vi "edit io channel.vi"(6 "user event":T2, 8 "error in":errorcluster, 9 "line":T1, 10 "engine configuration in":refnum<class "engine configuration.lvclass">, 11 "EthernetIP configuration in":refnum<class "EthernetIP configuration.lvclass">) -> (0 "error out":errorcluster, 2 "engine configuration out":refnum<class "engine configuration.lvclass">, 3 "EthernetIP configuration out":refnum<class "EthernetIP configuration.lvclass">)   [LabVIEW 2013, in "EthernetIP editor node.lvclass"]
uses:
  EthernetIP editor node.lvclass
  <vilib>/CEF_TreeControl/Node/UserEventRef.ctl
  <vilib>/CEF_TreeControl/Controls/EventCluster.ctl
  <vilib>/NI/Module Execution Interface/Engine Configuration/engine configuration.lvclass
  <vilib>/NI/TBM Modules/Ethernet IP/configuration/EthernetIP configuration.lvclass
  table line.ctl
  <vilib>/NI/TBM Modules/Ethernet IP/channel/EthernetIP Channel.lvclass
  <vilib>/NI/Tag Bus Module Framework/root configuration/TBM configuration.lvclass/TBM configuration.ctl
  <vilib>/NI/Tag Bus/tag/tag descriptor.lvclass/tag descriptor.ctl
  <vilib>/NI/Tag Bus Module Framework/root configuration/create GUID.vi
  <vilib>/CEF_TreeControl/NISE_CEF_TreeControl.lvlib
  <vilib>/NI/Tag Bus/tag/tag descriptor.lvclass
  <vilib>/NI/Tag Bus Module Framework/root configuration/TBM configuration.lvclass
  <vilib>/CEF_TreeControl/Node/NISE_CEF_Node.lvclass
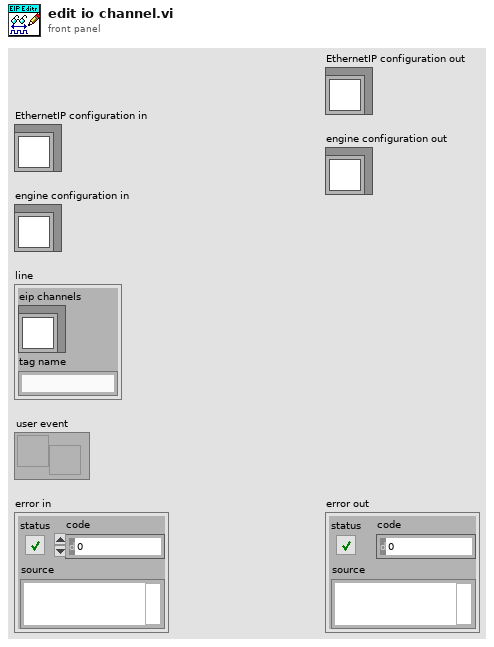
[diagram p1: front panel]
types:
  T1 = typedef "EthernetIP editor node.lvclass/table line.ctl" = cluster{"eip channels":refnum<class "EthernetIP Channel.lvclass">, "tag name":string}
  T2 = typedef "NISE_CEF_Node.lvclass/UserEventRef.ctl" = refnum<user-event>
  T3 = typedef "NISE_CEF_TreeControl.lvlib/EventCluster.ctl" = cluster{"command":string, "data":string}
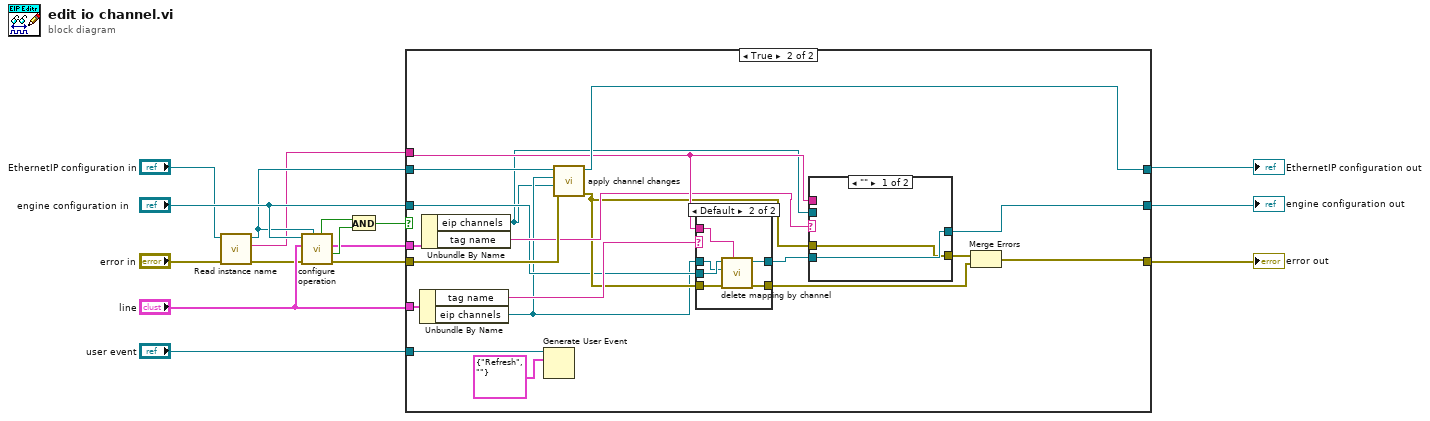
[diagram p0: block diagram]
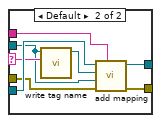
[diagram p3: hidden frame]
diagram:
  n1 = call <vilib>:"Read instance name.vi"("error in"="error in", "configuration in"="EthernetIP configuration in") -> ("error out"=w4:errorcluster, "instance id"=w1:string, "configuration out"=w2:refnum<class "EthernetIP configuration.lvclass">)  [unwired: 7 in]
  n2 = call "configure operation.vi"("EthernetIP configuration"=w2, "error in"=w4, "line item in"="line", "engine configuration in"="engine configuration in") -> ("error out"=w13:errorcluster, "success"=w16:bool, "line item out"=w6:T1, "changed"=w15:bool)  [unwired: 4 in]
  n3 = And(x=w15, y=w16) -> (x .and. y?=w12:bool)
  n4 = case shown="True" w12 {
    tunnel: [w18 w25] -> w9
    tunnel: [w19 w24] -> w10
    tunnel: "engine configuration in" -> [w19 w22]
    tunnel: w13 -> [w18 w36]
    tunnel: w6 -> [_ w33]
    tunnel: "line" -> [_ w37]
    tunnel: w2 -> [w17 w38]
    tunnel: [w17 w32] -> w8
    tunnel: w1 -> [_ w28]
    tunnel: "user event" -> [_ w34]
    frame False {
    }
    frame True {
      n5 = Unbundle By Name(w37) -> ("tag name"=w27:string, "eip channels"=w21:refnum<class "EthernetIP Channel.lvclass">)
      n6 = Unbundle By Name(w33) -> ("eip channels"=w20:refnum<class "EthernetIP Channel.lvclass">, "tag name"=w26:string)
      n7 = Generate User Event(user event=w34, event data cluster=T3 {"command"="Refresh", "data"=""} ("event data")) -> ()  [unwired: 2 in, 2 out]
      n8 = call <vilib>:"apply channel changes.vi"("error in"=w36, 9:"TBM channel in"=w20, 10:"TBM channel in"=w21, "EthernetIP configuration in"=w38) -> ("error out"=w23:errorcluster, "EthernetIP configuration out"=w32:refnum<class "EthernetIP configuration.lvclass">)  [unwired: 6 in]
      n9 = case shown="Default" w27 {
        tunnel: w28 -> [_ w56]
        tunnel: w22 -> [w50 w55]
        tunnel: [w50 w54] -> w31
        tunnel: [w49 w53] -> w30
        tunnel: w23 -> [w49 w52]
        tunnel: w21 -> [_ w51]
        frame "" {
        }
        frame Default {
          n10 = call <vilib>:"delete mapping by channel.vi"("owner ID"=w56, "error in"=w52, "channel"=w51, "engine configuration in"=w55) -> ("error out"=w53:errorcluster, "engine configuration out"=w54:refnum<class "engine configuration.lvclass">)  [unwired: 6 in]
        }
      }
      n11 = case shown="\"\"" w26 {
        selector: w26 -> [_ w42]
        tunnel: w31 -> [w40 w48]
        tunnel: [w40 w47] -> w24
        tunnel: [w39 w46] -> w29
        tunnel: w23 -> [w39 w45]
        tunnel: w28 -> [_ w44]
        tunnel: w20 -> [_ w41]
        frame "" {
        }
        frame Default {
          n12 = call <vilib>:"write tag name.vi"("name"=w42, "system tag in"=w41) -> ("system tag out"=w43:refnum<class "EthernetIP Channel.lvclass">)  [unwired: 8 in, 1 out]
          n13 = call <vilib>:"add mapping.vi"("owner ID"=w44, "error in"=w45, "channel"=w41, "tag descriptor"=w43, "engine configuration"=w48) -> ("error out"=w46:errorcluster, "engine configuration out"=w47:refnum<class "engine configuration.lvclass">)  [unwired: 5 in]
        }
      }
      n14 = Merge Errors(w29, w30) -> (w25:errorcluster)
    }
  }
  "engine configuration out" <- w10
  "EthernetIP configuration out" <- w8
  "error out" <- w9
